vi "Write Track.vi"(7 "Track Enable":T1, 8 "Error In":errorcluster, 9 "Write Position":i64, 10 "Audio In":T2, 11 "Track (File) References In":T3) -> (0 "Error Out":errorcluster, 3 "Track (File) References Out":T3)   [LabVIEW 2015]
doc: "Use this VI to write audio data to a Track file. This function will always write to both Left and Right channels. You must provide the VI with:\n\nTrack File References: Track Ref + Track Name. \n4-Track Audio: The data you want to write.\nTrack Enable: Define which tracks you want to write too. Setting to True will enable writes to this track. \nChannel Write Positions: Can specify a starting\\offset write position for each track you want to write too."
uses:
  Controls/Track (File) References.ctl
  Controls/Audio In.ctl
  Controls/Track Enable.ctl
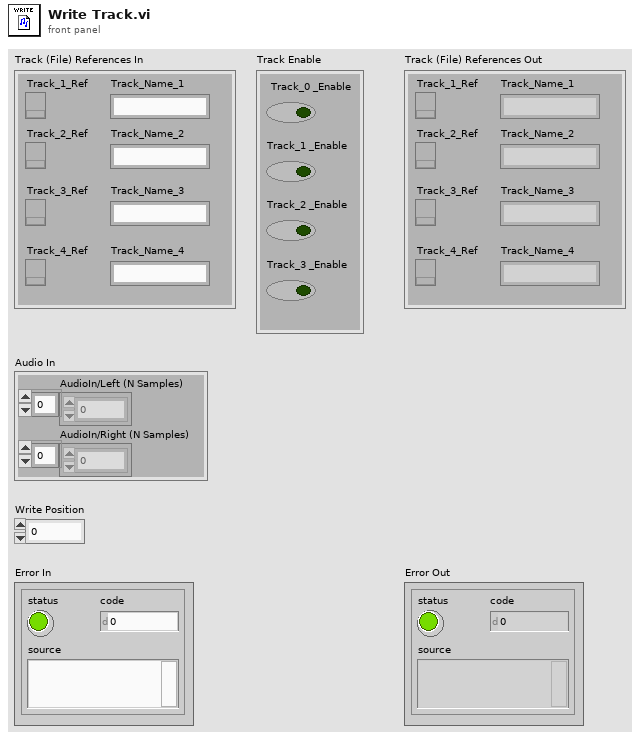
[diagram p1: front panel]
types:
  T1 = typedef "Track Enable.ctl" = cluster{"Track_0 _Enable ":bool, "Track_1 _Enable ":bool, "Track_2 _Enable ":bool, "Track_3 _Enable ":bool}
  T2 = typedef "Audio In.ctl" = cluster{"AudioIn/Left (N Samples)":i16[], "AudioIn/Right (N Samples)":i16[]}
  T3 = typedef "Track (File) References.ctl" = cluster{"Track_1_Ref":refnum<k34>, "Track_2_Ref":refnum<k34>, "Track_3_Ref":refnum<k34>, "Track_4_Ref":refnum<k34>, "Track_Name_1":string, "Track_Name_2":string, "Track_Name_3":string, "Track_Name_4":string}
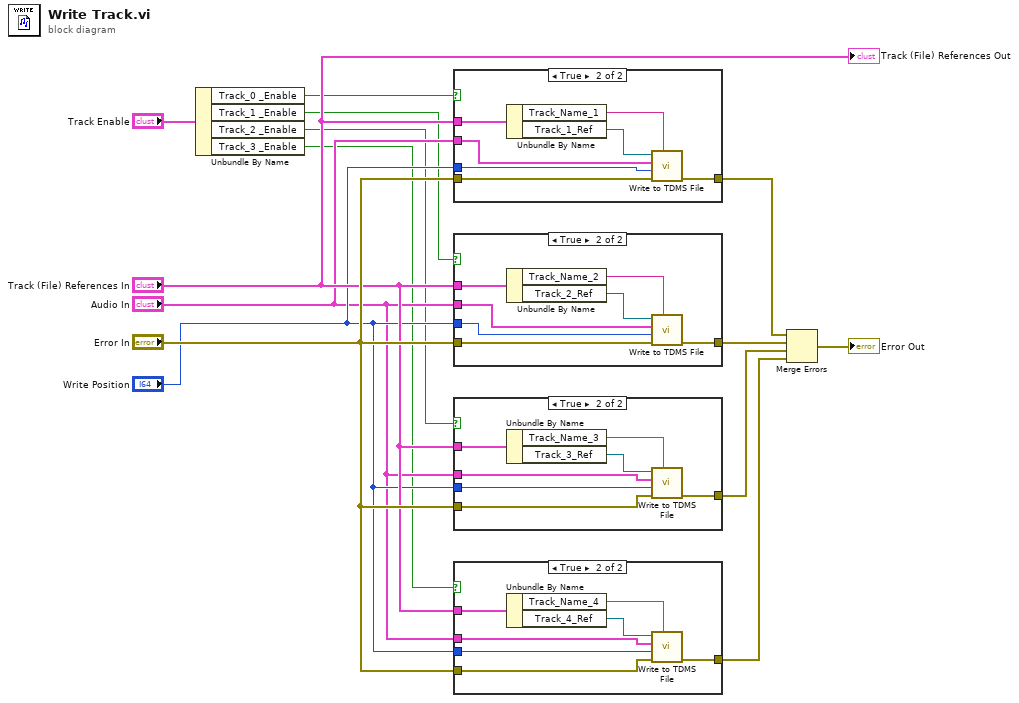
[diagram p0: block diagram]
diagram:
  n1 = Unbundle By Name("Track Enable") -> ("Track_0 _Enable"=w5:bool, "Track_1 _Enable"=w4:bool, "Track_2 _Enable"=w3:bool, "Track_3 _Enable"=w2:bool)
  n2 = case shown="True" w5 {
    tunnel: "Track (File) References In" -> [_ w22]
    tunnel: "Error In" -> [w15 w18]
    tunnel: [w15 w19] -> w12
    tunnel: "Write Position" -> [_ w17]
    tunnel: "Audio In" -> [_ w16]
    frame False {
    }
    frame True {
      n3 = Unbundle By Name(w22) -> ("Track_Name_1"=w21:string, "Track_1_Ref"=w20:refnum<k34>)
      n4 = call "Write to TDMS File.vi"("Track Name"=w21, "Error In"=w18, "Write Position"=w17, "Audio In"=w16, "TDMS Reference In"=w20) -> ("Error Out"=w19:errorcluster)  [unwired: 5 in, 1 out]
    }
  }
  n5 = case shown="True" w4 {
    tunnel: "Track (File) References In" -> [_ w30]
    tunnel: "Error In" -> [w23 w26]
    tunnel: [w23 w29] -> w11
    tunnel: "Write Position" -> [_ w25]
    tunnel: "Audio In" -> [_ w24]
    frame False {
    }
    frame True {
      n6 = Unbundle By Name(w30) -> ("Track_Name_2"=w28:string, "Track_2_Ref"=w27:refnum<k34>)
      n7 = call "Write to TDMS File.vi"("Track Name"=w28, "Error In"=w26, "Write Position"=w25, "Audio In"=w24, "TDMS Reference In"=w27) -> ("Error Out"=w29:errorcluster)  [unwired: 5 in, 1 out]
    }
  }
  n8 = case shown="True" w3 {
    tunnel: "Track (File) References In" -> [_ w38]
    tunnel: "Error In" -> [w31 w34]
    tunnel: [w31 w37] -> w10
    tunnel: "Write Position" -> [_ w33]
    tunnel: "Audio In" -> [_ w32]
    frame False {
    }
    frame True {
      n9 = Unbundle By Name(w38) -> ("Track_Name_3"=w36:string, "Track_3_Ref"=w35:refnum<k34>)
      n10 = call "Write to TDMS File.vi"("Track Name"=w36, "Error In"=w34, "Write Position"=w33, "Audio In"=w32, "TDMS Reference In"=w35) -> ("Error Out"=w37:errorcluster)  [unwired: 5 in, 1 out]
    }
  }
  n11 = case shown="True" w2 {
    tunnel: "Track (File) References In" -> [_ w46]
    tunnel: "Error In" -> [w39 w42]
    tunnel: [w39 w45] -> w9
    tunnel: "Write Position" -> [_ w41]
    tunnel: "Audio In" -> [_ w40]
    frame False {
    }
    frame True {
      n12 = Unbundle By Name(w46) -> ("Track_Name_4"=w44:string, "Track_4_Ref"=w43:refnum<k34>)
      n13 = call "Write to TDMS File.vi"("Track Name"=w44, "Error In"=w42, "Write Position"=w41, "Audio In"=w40, "TDMS Reference In"=w43) -> ("Error Out"=w45:errorcluster)  [unwired: 5 in, 1 out]
    }
  }
  n14 = Merge Errors(w12, w11, w10, w9) -> (→"Error Out":errorcluster)
  "Track (File) References Out" <- "Track (File) References In"
